vi "channel_enable_ASIC_v2.vi"(8 "error in":errorcluster, 10 "Channel Combination":u32=9764, 11 "Connection ID in":refnum<k5>) -> (0 "error out":errorcluster, 3 "Connection ID out":refnum<k5>)   [LabVIEW 2009]
panel:
  out "data read value":u32=72
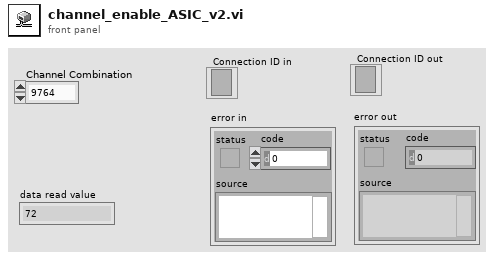
[diagram p1: front panel]
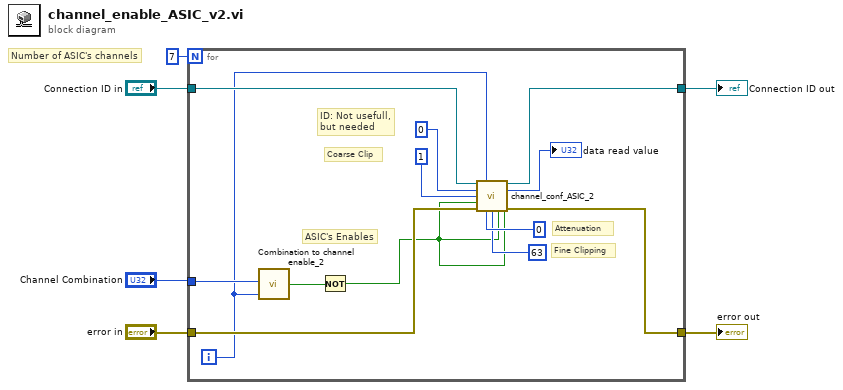
[diagram p0: block diagram]
diagram:
  # "Number of ASIC's channels"
  n1 = for {
    N: 7 -> [_]
    tunnel: "Channel Combination" -> [w19]
    tunnel: "error in" -> [w13]
    tunnel: [w12] -> w3
    tunnel: [w11] -> w1
    tunnel: "Connection ID in" -> [w14]
    i -> [w9]
    # "ASIC's Enables"
    # "Attenuation"
    # "Fine Clipping"
    # "Coarse Clip"
    # "ID: Not usefull,\nbut needed"
    n2 = call "Combination to channel enable_2.vi"("Channel"=w9, "Channel Combination"=w19) -> ("Enable"=w8:bool)  [unwired: 1 in]
    n3 = Not(x=w8) -> (.not. x?=w7:bool)
    n4 = call "channel_conf_ASIC_2.vi"("connection ID"=w14, "Ring"=w9, "Id in"=u32 0, "Clip_sel_b"=u32 1, "CompBuf_en_b"=w7, "error out"=w13, "Att gain"=u32 0, "Ib_ClipVb"=u32 63, "Clip_en_b"=w7, "Att_en_b"=w7) -> ("connection ID out"=w11:refnum<k5>, "data read value"=→"data read value":u32, "error out 2"=w12:errorcluster)  [unwired: 1 in, 2 out]
  }
  "error out" <- w3
  "Connection ID out" <- w1
